vi "Error Engine.vi"(8 "error in":errorcluster) -> (0 "error out":errorcluster)   [LabVIEW 2023, in "HardwareAbstractionLayer_LVOOP.lvlib" / "Error Handler.lvclass"]
uses:
  Error Handler.lvclass
  Control/Error Data.ctl
  Control/Error_States.ctl
  Control/Error File.ctl
  Control/Error and Event Log.ctl
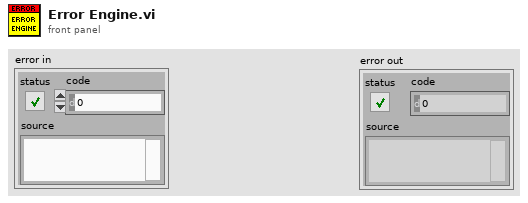
[diagram p1: front panel]
types:
  T1 = typedef "HardwareAbstractionLayer_LVOOP.lvlib/Error Handler.lvclass/Error File.ctl" = enum16{"Open", "Read File", "Write File", "Close"}
  T2 = typedef "HardwareAbstractionLayer_LVOOP.lvlib/Error Handler.lvclass/Error Data.ctl" = cluster{"Data":variant, "States":T3}
  T3 = typedef "HardwareAbstractionLayer_LVOOP.lvlib/Error Handler.lvclass/Error_States.ctl" = enum16{"No Error", "Error_Log", "Event_Log"}
  T4 = typedef "HardwareAbstractionLayer_LVOOP.lvlib/Error Handler.lvclass/Error and Event Log.ctl" = cluster{"Error/Event Log":string, "TimeStamp":string, "VI Source Name":string, "Description ":string}
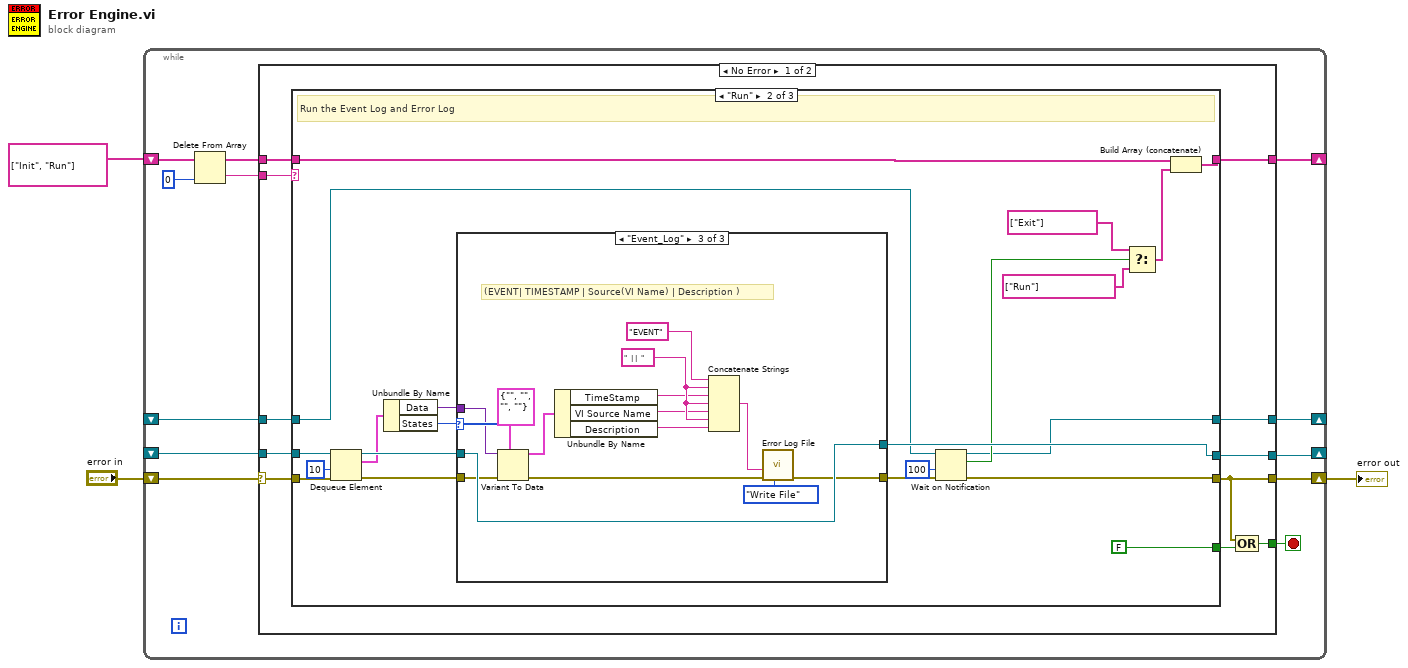
[diagram p0: block diagram]
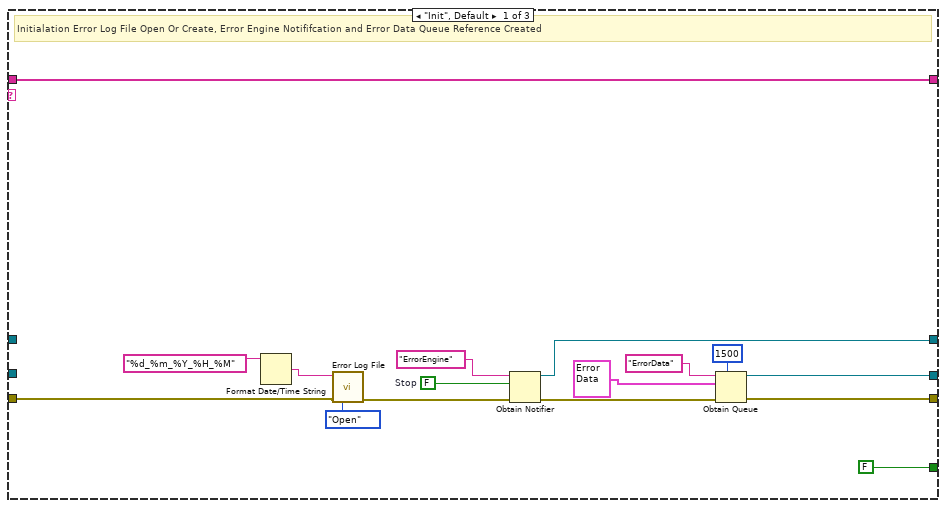
[diagram p2: hidden frame]
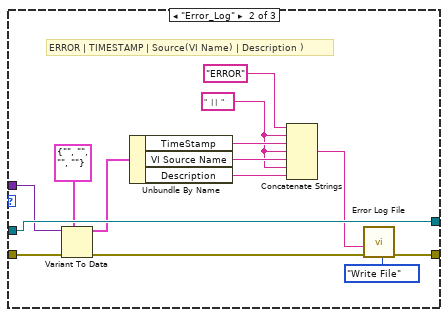
[diagram p4: hidden frame]
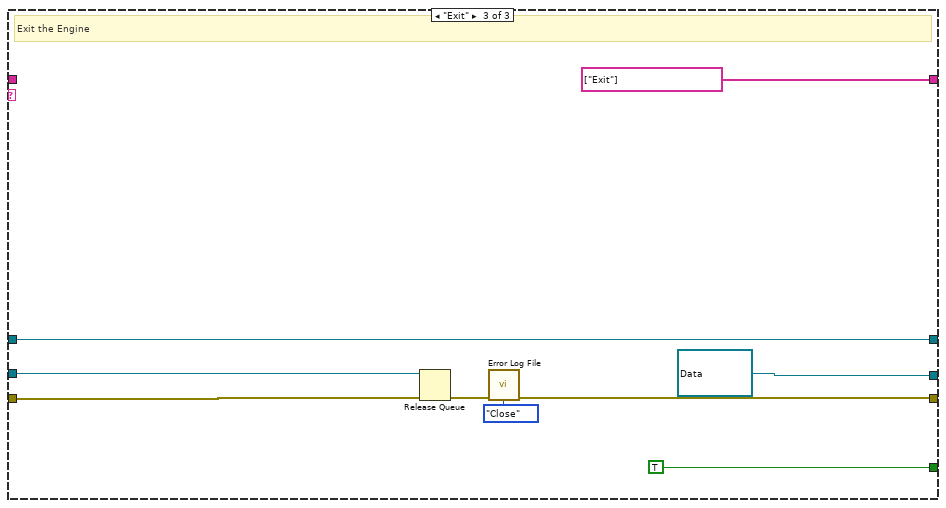
[diagram p5: hidden frame]
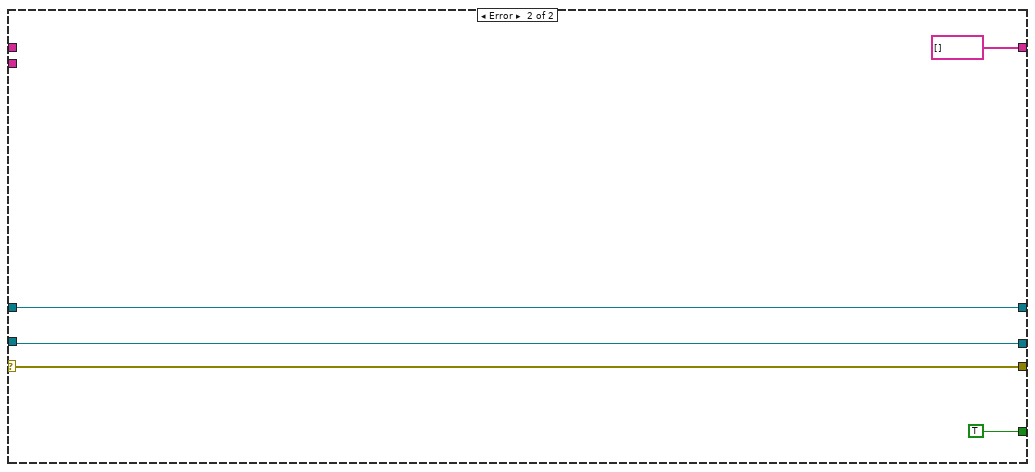
[diagram p6: hidden frame]
diagram:
  n1 = while {
    shift-right: [w10] -> _
    shift-left: string[] ["Init", "Run"] -> [w14]
    shift-right: [w9] -> _
    shift-left: _ -> [w15]
    shift-right: [w7] -> w1
    shift-left: "error in" -> [w4]
    shift-right: [w5] -> _
    shift-left: _ -> [w6]
    stop <- w8 stop-if-true
    n2 = Delete From Array(array=w14, index=0) -> (deleted portion=w13:string, array with subset deleted=w11:string[])  [unwired: 1 in]
    n3 = case shown="No Error" w4 {
      selector: w4 -> [w25 w106]
      tunnel: w15 -> [w26 w105]
      tunnel: w13 -> [w24 _]
      tunnel: w11 -> [w23 _]
      tunnel: [w22 string[] []] -> w10
      tunnel: [w21 w105] -> w9
      tunnel: [w19 TRUE] -> w8
      tunnel: [w18 w106] -> w7
      tunnel: w6 -> [w17 w103]
      tunnel: [w16 w103] -> w5
      frame No Error {
        n4 = case shown="\"Run\"" w24 {
          tunnel: w26 -> [_ w63 w96]
          tunnel: w25 -> [w29 w62 w97]
          tunnel: w23 -> [w42 w56 _]
          tunnel: [w30 w57 refnum<queue> refnum ("queue out")] -> w21
          tunnel: [w28 w48 w95] -> w18
          tunnel: [w42 w54 string[] ["Exit"]] -> w22
          tunnel: [FALSE FALSE TRUE] -> w20
          tunnel: w17 -> [_ w47 w100]
          tunnel: [w31 w44 w100] -> w16
          frame "Init", Default {
            w38 = FALSE  # Stop
            # "Initialation Error Log File Open Or Create, Error Engine Notififcation and Error Data Queue Reference Created"
            n5 = Format Date/Time String(time format string (%c)="%d_%m_%Y_%H_%M") -> (date/time string=w27:string)  [unwired: 2 in]
            n6 = call "Error Log File.vi"("error in"=w29, "File Options"=Error_File."Open", "File Name"=w27) -> ("error out"=w32:errorcluster)  [unwired: 7 in, 1 out]
            n7 = Obtain Notifier(name (unnamed)="ErrorEngine", notification data type=w38, error in (no error)=w32) -> (notifier out=w31:refnum<notifier>, error out=w36:errorcluster)  [unwired: 1 in, 1 out]
            n8 = Obtain Queue(max queue size (-1, unlimited)=1500, name (unnamed)="ErrorData", element data type=T2 {"Data"=variant, "States"=enum."Event_Log"} ("Data"), error in (no error)=w36) -> (queue out=w30:refnum<queue>, error out=w28:errorcluster)  [unwired: 1 in, 1 out]
          }
          frame "Run" {
            # "Run the Event Log and Error Log"
            n9 = Dequeue Element(queue=w63, timeout in ms (-1)=10, error in (no error)=w62) -> (queue out=w61:refnum<queue>, element=w60:T2, error out=w59:errorcluster)  [unwired: 1 out]
            n10 = Unbundle By Name(w60) -> ("Data"=w53:variant, "States"=w58:T3)
            n11 = case shown="\"Event_Log\"" w58 {
              tunnel: w61 -> [w65 w79 w93]
              tunnel: w59 -> [w64 w76 w92]
              tunnel: [w65 w79 w93] -> w57
              tunnel: [w64 w70 w88] -> w49
              tunnel: w53 -> [_ w78 w91]
              frame "No Error", Default {
              }
              frame "Error_Log" {
                w72 = "  | |  " ("string")
                # "ERROR | TIMESTAMP | Source(VI Name) | Description )"
                n12 = Variant To Data(error in=w76, type=T4 {"Error/Event Log"="", "TimeStamp"="", "VI Source Name"="", "Description "=""} ("Error and Event Log"), Variant=w78) -> (data=w75:T4, error out=w68:errorcluster)
                n13 = Unbundle By Name(w75) -> ("TimeStamp"=w74:string, "VI Source Name"=w73:string, "Description"=w71:string)
                n14 = Concatenate Strings("ERROR" ("string"), w72, w74, w72, w73, w72, w71) -> (w66:string)
                n15 = call "Error Log File.vi"("error in"=w68, "Write"=w66, "File Options"=Error_File."Write File") -> ("error out"=w70:errorcluster)  [unwired: 7 in, 1 out]
              }
              frame "Event_Log" {
                w87 = "  | |  " ("string")
                # "(EVENT| TIMESTAMP | Source(VI Name) | Description )"
                n16 = Variant To Data(error in=w92, type=T4 {"Error/Event Log"="", "TimeStamp"="", "VI Source Name"="", "Description "=""} ("Error and Event Log"), Variant=w91) -> (data=w89:T4, error out=w81:errorcluster)
                n17 = Unbundle By Name(w89) -> ("TimeStamp"=w86:string, "VI Source Name"=w85:string, "Description"=w84:string)
                n18 = Concatenate Strings("EVENT" ("string"), w87, w86, w87, w85, w87, w84) -> (w83:string)
                n19 = call "Error Log File.vi"("error in"=w81, "Write"=w83, "File Options"=Error_File."Write File") -> ("error out"=w88:errorcluster)  [unwired: 7 in, 1 out]
              }
            }
            n20 = Wait on Notification(notifier=w47, timeout in ms (-1)=100, error in (no error)=w49) -> (notifier out=w44:refnum<notifier>, notification=w45:bool, error out=w48:errorcluster)  [unwired: 1 in, 1 out]
            n21 = Select(t=string[] ["Exit"] ("f"), s=w45, f=string[] ["Run"] ("array")) -> (s? t:f=w52:string[])
            n22 = Build Array (concatenate)(w56, w52) -> (w54:string[])
          }
          frame "Exit" {
            # "Exit the Engine"
            n23 = Release Queue(queue=w96, error in (no error)=w97) -> (error out=w98:errorcluster)  [unwired: 1 in, 2 out]
            n24 = call "Error Log File.vi"("error in"=w98, "File Options"=Error_File."Close") -> ("error out"=w95:errorcluster)  [unwired: 8 in, 1 out]
          }
        }
        n25 = Compound Arithmetic op=OR(w18, w20) -> (w19:bool)
      }
      frame Error {
      }
    }
  }
  "error out" <- w1
